vi "diagram.vi"() -> ()   [LabVIEW 2024]
uses:
  <vilib>/Analysis/NI_AALPro.lvlib
panel:
  in  "index (row)":i32=2
  out "error":i32
  out "interpolation error":dbl format="%0.2f"
  out "interpolation value":dbl format="%0.2f"
  out "XY Graph":cluster{dbl[], dbl[]}[](graph)
  out "Table Control":string[][](table)
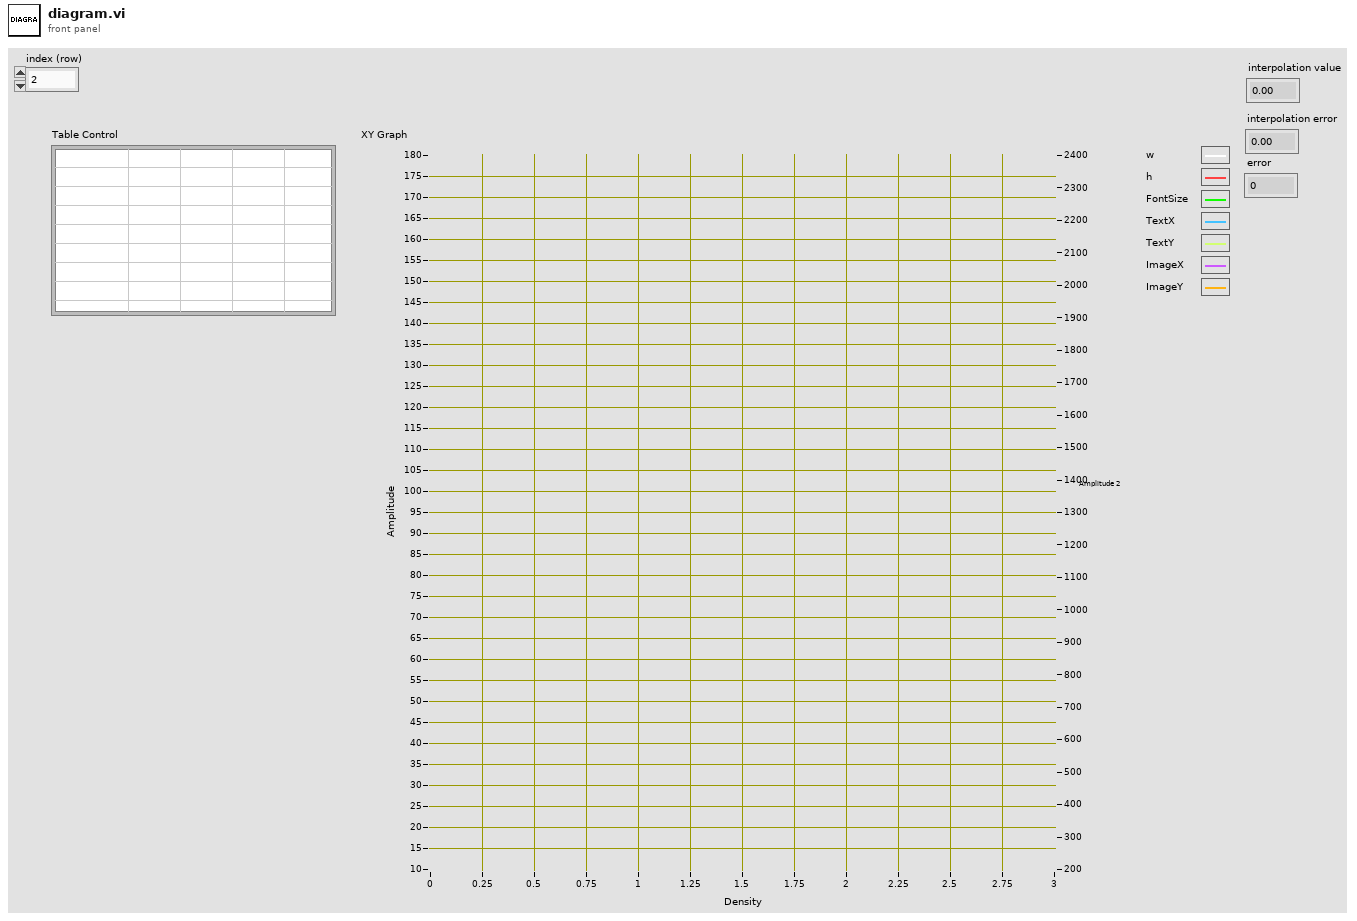
[diagram p1: front panel]
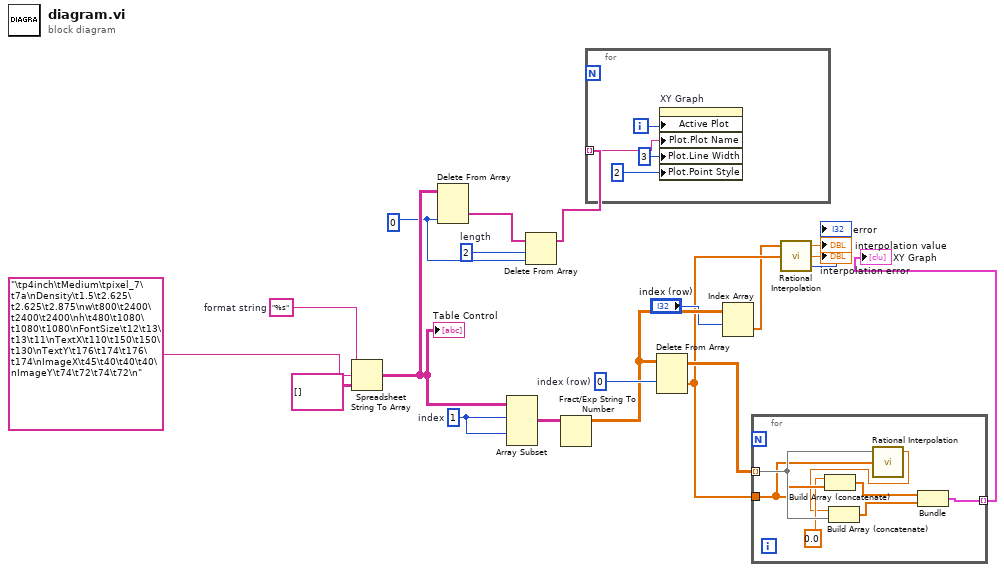
[diagram p0: block diagram]
diagram:
  w6 = 2  # length
  w7 = 0
  w15 = 0  # index (row)
  w17 = 1  # index
  w19 = "%s"  # format string
  n1 = Spreadsheet String To Array(format string=w19, spreadsheet string="\tp4inch\tMedium\tpixel_7\t7a\nDensity\t1.5\t2.625\t2.625\t2.875\nw\t800\t2400\t2400\t2400\nh\t480\t1080\t1080\t1080\nFontSize\t12\t13\t13\t11\nTextX\t110\t150\t150\t130\nTextY\t176\t174\t176\t174\nImageX\t45\t40\t40\t40\nImageY\t74\t72\t74\t72\n", array type (2D Dbl)=string[][] []) -> (array=w10:string[][])  [unwired: 1 in]
  "Table Control" <- w10
  n2 = Delete From Array(array=w10, index (col)=w7) -> (deleted portion=w9:string[])  [unwired: 2 in, 1 out]
  n3 = Array Subset(array=w10, index (row)=w17, index (col)=w17) -> (w16:string[][])  [unwired: 2 in]
  n4 = Delete From Array(array=w9, length=w6, index=w7) -> (array with subset deleted=w8:string[])  [unwired: 1 out]
  n5 = Fract/Exp String To Number(string=w16) -> (number=w14:dbl[][])  [unwired: 3 in, 1 out]
  n6 = for {
    tunnel: w8 -> [w23] mode=indexing
    i -> [w24]
    n7 = property on="XY Graph" class="XYGraph (strict)"("Active Plot"=w24, "Plot.Plot Name"=w23, "Plot.Line Width"=u8 3, "Plot.Point Style"=u8 2) -> ()  [unwired: 2 in, 2 out]
  }
  n8 = Delete From Array(array=w14, index (row)=w15) -> (deleted portion=w5:dbl[], array with subset deleted=w12:dbl[][])  [unwired: 2 in]
  n9 = Index Array(array=w14, index (row)="index (row)") -> (element=w4:dbl[])  [unwired: 1 in]
  n10 = for {
    tunnel: w12 -> [w30] mode=indexing
    tunnel: w5 -> [w27]
    tunnel: [w31] -> w11 mode=indexing
    n11 = Build Array (concatenate)(0.0, w27) -> (w28:dbl[])
    n12 = call <vilib>:"Rational Interpolation.vi"("X"=w27, "Y"=w30) -> ("interpolation value"=w25:dbl)  [unwired: 1 in, 2 out]
    n13 = Build Array (concatenate)(w25, w30) -> (w29:dbl[])
    n14 = Bundle(w28, w29) -> (w31:cluster{dbl[], dbl[]})  [unwired: 1 in]
  }
  "XY Graph" <- w11
  n15 = call <vilib>:"Rational Interpolation.vi"("X"=w5, "Y"=w4) -> ("error"=→"error":i32, "interpolation error"=→"interpolation error":dbl, "interpolation value"=→"interpolation value":dbl)  [unwired: 1 in]
